vi "Time.TimeStamp to String.vi"(7 "TimeFormat":T1, 11 "Time Stamp in":timestamp) -> (3 "Time String Out":string)   [LabVIEW 2024]
uses:
  Time.Format Selector.ctl
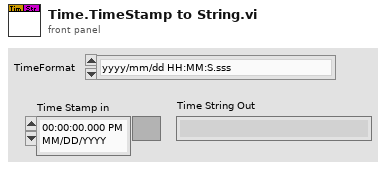
[diagram p1: front panel]
types:
  T1 = typedef "Time.Format Selector.ctl" = enum16{"yyyy/mm/dd HH:MM:S.sss", "yyyy/mm/dd HH:MM:SS", "yyyy-MM-ddTHH:mm:ss[.mmm]", "YYYYMMDD_HHMMSS"}
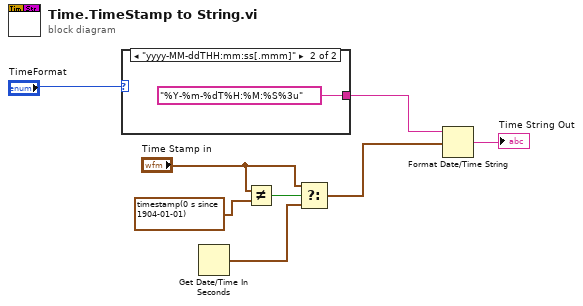
[diagram p0: block diagram]
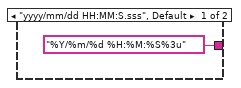
[diagram p2: hidden frame]
diagram:
  n1 = case shown="\"yyyy-MM-ddTHH:mm:ss[.mmm]\"" "TimeFormat" {
    tunnel: ["%Y/%m/%d %H:%M:%S%3u" ("time format string (%c)") "%Y-%m-%dT%H:%M:%S%3u" ("time format string (%c)")] -> w1
    frame "yyyy/mm/dd HH:MM:S.sss", Default {
    }
    frame "yyyy-MM-ddTHH:mm:ss[.mmm]" {
    }
  }
  n2 = Get Date/Time In Seconds() -> (seconds since 1Jan1904=w4:timestamp)
  n3 = Not Equal?(x="Time Stamp in", y=timestamp(0 s since 1904-01-01) ("Time Stamp in")) -> (x != y?=w6:bool)
  n4 = Select(t="Time Stamp in", s=w6, f=w4) -> (s? t:f=w3:timestamp)
  n5 = Format Date/Time String(time format string (%c)=w1, seconds (now)=w3) -> (date/time string=→"Time String Out":string)  [unwired: 1 in]
